vi "Counter - Count Edges (Continuous Clock).vi"() -> ()   [LabVIEW 2017]
doc: "本范例演示连续读回所有经计数器输入计算到的数字边沿的方法。 本范例采用外部时钟，从而计数寄存器采样按固定间隔进行。 如不需要实现计数寄存器确定性采样，请参考不采用外部时钟的Count Edges范例。\n\n关于将信号连接至DAQ设备的方法，可参考设备文档。"
uses:
  <vilib>/Utility/error.llb/DialogType.ctl
  <vilib>/DAQmx/read.llb/DAQmx Read (Counter 1D U32 1Chan NSamp).vi
  <vilib>/DAQmx/create/channels.llb/DAQmx Create Channel (CI-Count Edges).vi
  <vilib>/DAQmx/configure/timing.llb/DAQmx Timing (Sample Clock).vi
  <vilib>/DAQmx/miscellaneous.llb/DAQmx Fill In Error Info.vi
  <resource>/objmgr/daqmx.rc
panel:
  in  "有效边沿":i32(ring)=10280 items=["上升"=10280, "下降"=10171]
  in  "触发类型":T1(tab)
  in  "边沿":i32(ring)=10280 items=["上升"=10280, "下降"=10171]
  in  "数字触发源":tag
  in  "暂停条件":i32(ring)=10192 items=["高"=10192, "低"=10214]
  in  "暂停触发源":tag
  in  "计数重置接线端":tag
  in  "边沿":i32(ring)=10280 items=["上升"=10280, "下降"=10171]
  out "数据":u32[](array[numeric])
  in  "输入接线端":tag="PFI8"
  in  "计数器":tag="Dev1/ctr0"
  in  "停止":bool
  in  "每次循环采样数":i32=100
  in  "采样率":dbl=1000.0
  in  "采样时钟源":tag="PFI0"
  # "通道设置"
  # "采集数据"
  # "定时设置"
  # "触发设置"
  # "如需配置并使用触发/计数重置，必须先在上面选择相应的选项卡。  有些硬件不支持上述选项－更多信息见设备的相应文档。"
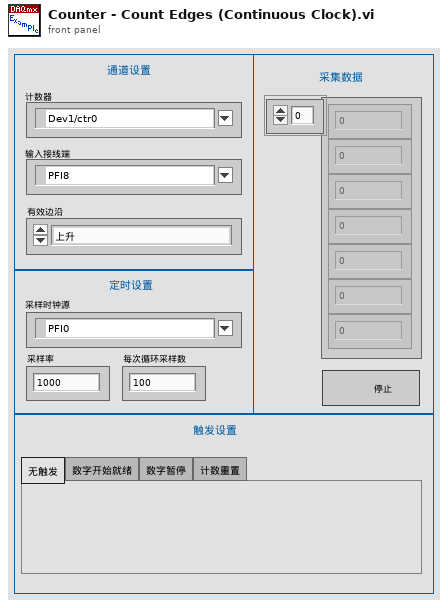
[diagram p1: front panel]
types:
  T1 = enum32{"No Trigger", "Digital Arm Start", "Digital Pause", "Count Reset"}
  T2 = typedef "DialogType.ctl" = u16
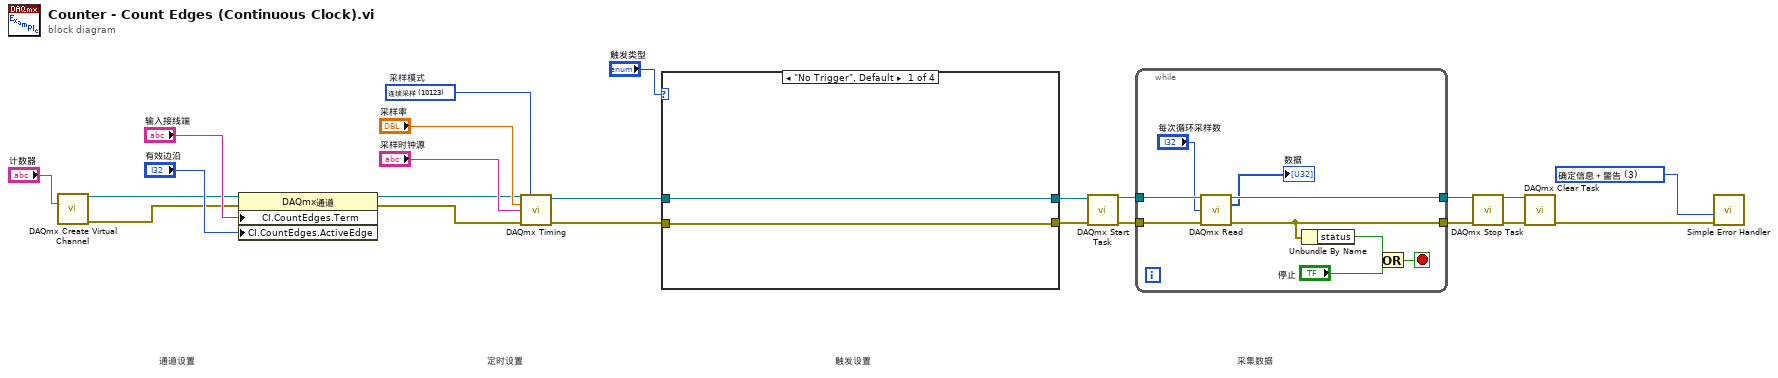
[diagram p0: block diagram]
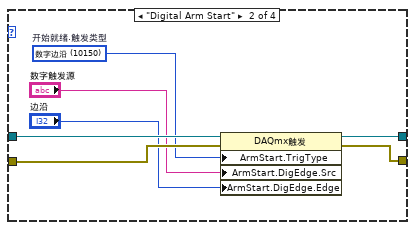
[diagram p2: hidden frame]
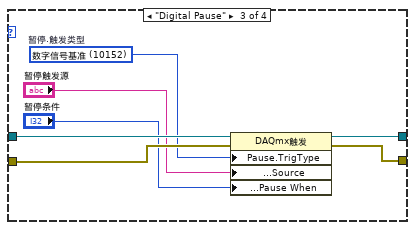
[diagram p3: hidden frame]
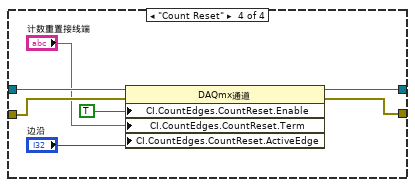
[diagram p4: hidden frame]
diagram:
  w1 = T2 3 items=["无对话框", "确定信息", "继续或停止信息", "确定信息＋警告", "继续/停止＋警告"] ("对话框类型（确定信息：1）")
  w21 = 10123 items=["有限采样"=10178, "连续采样"=10123, "硬件定时单点"=12522]  # 采样模式
  # "采集数据"
  # "触发设置"
  # "定时设置"
  # "通道设置"
  n1 = call-poly <vilib>:"DAQmx Create Virtual Channel.vi"("counter"="计数器") -> ("task out"=w14:refnum<k21>, "error out"=w11:errorcluster)  [unwired: 13 in]
  n2 = property class="DAQmx通道"(reference=w14, error in=w11, "CI.CountEdges.Term"="输入接线端", "CI.CountEdges.ActiveEdge"="有效边沿") -> (reference out=w13:refnum<k21>, error out=w12:errorcluster)
  n3 = call-poly <vilib>:"DAQmx Timing.vi"("task/channels in"=w13, "sample mode"=w21, "rate"="采样率", "source"="采样时钟源", "error in"=w12) -> ("task out"=w7:refnum<k21>, "error out"=w6:errorcluster)  [unwired: 9 in]
  n4 = case shown="\"No Trigger\", Default" "触发类型" {
    tunnel: w7 -> [w25 w32 w39 w46]
    tunnel: w6 -> [w24 w29 w36 w43]
    tunnel: [w25 w31 w38 w45] -> w8
    tunnel: [w24 w30 w37 w44] -> w9
    frame "No Trigger", Default {
    }
    frame "Digital Arm Start" {
      w26 = 10150 items=["数字边沿"=10150, "无"=10230]  # 开始就绪.触发类型
      n5 = property class="DAQmx触发"(reference=w32, error in=w29, "ArmStart.TrigType"=w26, "ArmStart.DigEdge.Src"="数字触发源", "ArmStart.DigEdge.Edge"="边沿") -> (reference out=w31:refnum<k21>, error out=w30:errorcluster)
    }
    frame "Digital Pause" {
      w35 = 10152 items=["模拟信号基准"=10101, "模拟窗"=10103, "数字信号基准"=10152, "数字模式"=10398, "无"=10230]  # 暂停.触发类型
      n6 = property class="DAQmx触发"(reference=w39, error in=w36, "Pause.TrigType"=w35, "More:Pause:Digital Level:Source"="暂停触发源", "More:Pause:Digital Level:Pause When"="暂停条件") -> (reference out=w38:refnum<k21>, error out=w37:errorcluster)
    }
    frame "Count Reset" {
      n7 = property class="DAQmx通道"(reference=w46, error in=w43, "CI.CountEdges.CountReset.Enable"=TRUE ("计数器输入.边沿计数.计数重置.启用"), "CI.CountEdges.CountReset.Term"="计数重置接线端", "CI.CountEdges.CountReset.ActiveEdge"="边沿") -> (reference out=w45:refnum<k21>, error out=w44:errorcluster)
    }
  }
  n8 = call <vilib>:"DAQmx Start Task.vi"("task/channels in"=w8, "error in"=w9) -> ("task out"=w20:refnum<k21>, "error out"=w19:errorcluster)  [unwired: 12 in]
  n9 = while {
    tunnel: w20 -> [w55]
    tunnel: w19 -> [w54]
    tunnel: [w51] -> w4
    tunnel: [w52] -> w5
    stop <- w53 stop-if-true
    n10 = call-poly <vilib>:"DAQmx Read.vi"("task/channels in"=w55, "number of samples per channel"="每次循环采样数", "error in"=w54) -> ("task out"=w52:refnum<k21>, "data"=→"数据":u32[], "error out"=w51:errorcluster)  [unwired: 10 in]
    n11 = Unbundle By Name(w51) -> ("status"=w50:bool)
    n12 = Or(x=w50, y="停止") -> (x .or. y?=w53:bool)
  }
  n13 = call <vilib>:"DAQmx Stop Task.vi"("task/channels in"=w5, "error in"=w4) -> ("task out"=w2:refnum<k21>, "error out"=w3:errorcluster)  [unwired: 12 in]
  n14 = call <vilib>:"DAQmx Clear Task.vi"("task in"=w2, "error in"=w3) -> ("error out"=w18:errorcluster)  [unwired: 13 in]
  n15 = call <vilib>:"Simple Error Handler.vi"("type of dialog (OK msg:1)"=w1, "error in (no error)"=w18) -> ()  [unwired: 3 in, 5 out]
